vi "tt-钩外多胶检测-kA.vi"(9 "镜像产品角度":dbl=45.0, 11 "ImageSrc":T1(plugin-control)) -> (3 "ImgOut":T1(plugin-control))   [LabVIEW 2018]
uses:
  <vilib>/vision/Image Controls.llb/IMAQ Image.ctl
  <vilib>/vision/NI_Vision_Development_Module.lvlib
panel:
  out "error out":errorcluster
  out "Image Dst Out":T1
  in  "钩端向上部偏移量":dbl=100.0
  in  "Annulus":T2={"Center X"=0, "Center Y"=0, "Inner Radius"=27, "Outer Radius"=107, "Start Angle"=0.0, "End Angle"=0.0} {"End Angle" min=-90.0 max=90.0 step=1.0 format="%.2f"; "Start Angle" min=-90.0 max=90.0 step=1.0 format="%.2f"; "Center X" scale=0.0..1024.0}
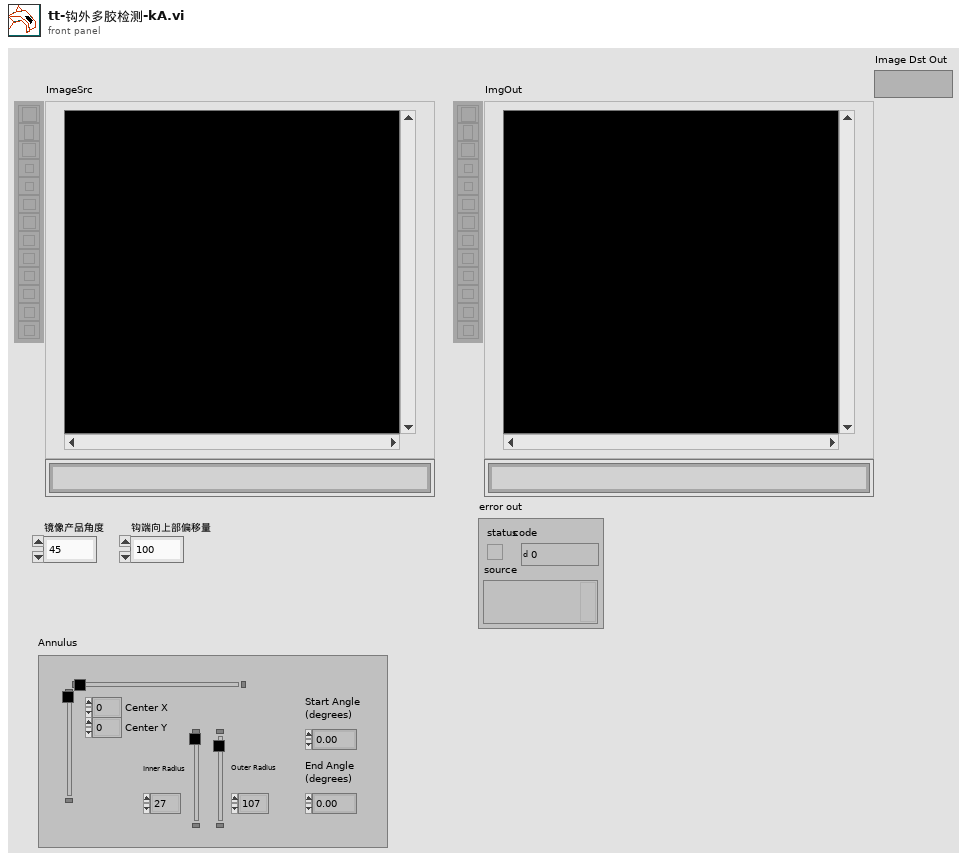
[diagram p1: front panel]
types:
  T1 = typedef "IMAQ Image.ctl" = refnum<image>
  T2 = typedef "IMAQ Circle" = cluster{"Center X":i32, "Center Y":i32, "Inner Radius":i32, "Outer Radius":i32, "Start Angle":dbl, "End Angle":dbl}
  T3 = typedef "Image Type" = u32
  T4 = typedef "ROI Descriptor" = cluster{"Global Rectangle":i32[], "Contours":cluster{"ID":enum32{"External", "Internal"}, "Type":u32, "Coordinates":i32[]}[]}
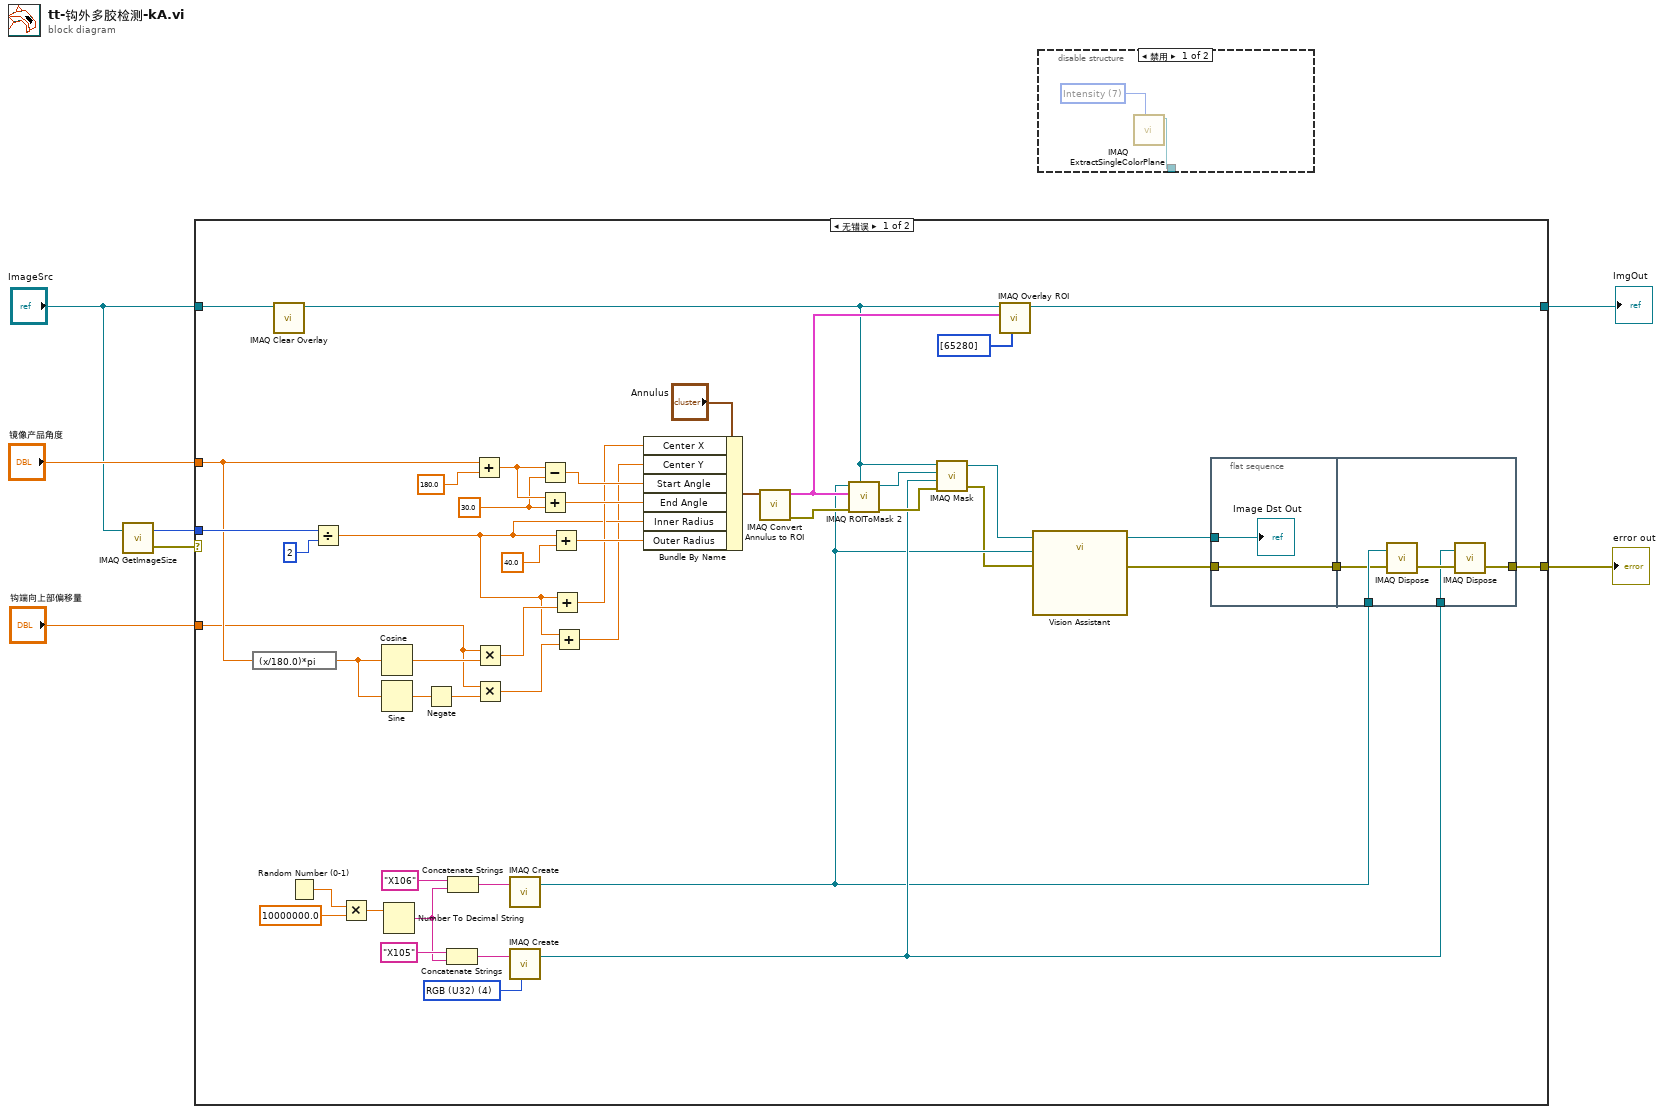
[diagram p0: block diagram]
diagram:
  n1 = call "IMAQ GetImageSize"("Image"="ImageSrc") -> ("Y Resolution"=w4:i32, "error out"=w5:errorcluster)  [unwired: 3 in, 1 out]
  n2 = case shown="无错误" w5 {
    selector: w5 -> [_ w62]
    tunnel: "镜像产品角度" -> [w43 _]
    tunnel: "ImageSrc" -> [w20 w63]
    tunnel: w4 -> [w47 _]
    tunnel: "钩端向上部偏移量" -> [w38 _]
    tunnel: [w29 w63] -> w2
    tunnel: [w15 w62] -> w1
    frame No Error {
      w16 = T3 4 items=["Grayscale (U8)", "Grayscale (I16)", "Grayscale (SGL)", "Complex (CSG)", "RGB (U32)", "HSL (U32)", "RGB (U64)", "Grayscale (U16)"] ("Image Type")
      w48 = 30.0 ("y")
      n3 = expression code="(x/180.0)*pi" ("角度转换至弧度")(w43) -> (w41:dbl)
      n4 = call "IMAQ Clear Overlay"("Image"=w20) -> ("Image Out"=w19:T1)  [unwired: 9 in, 1 out]
      n5 = Random Number (0-1)() -> (number: 0 to 1=w23:dbl)
      n6 = Divide(x=w47, y=2) -> (x/y=w34:dbl)
      n7 = Multiply(x=w23, y=10000000.0) -> (x*y=w25:dbl)
      n8 = Cosine(x=w41) -> (cos(x)=w40:dbl)
      n9 = Sine(x=w41) -> (sin(x)=w42:dbl)
      n10 = Number To Decimal String(number=w25) -> (decimal integer string=w22:string)  [unwired: 1 in]
      n11 = Negate(x=w42) -> (-x=w39:dbl)
      n12 = Concatenate Strings("X105" ("字符串"), w22) -> (w27:string)
      n13 = Concatenate Strings("X106" ("字符串"), w22) -> (w30:string)
      n14 = Add(x=w43, y=180.0) -> (x+y=w51:dbl)
      n15 = Multiply(x=w38, y=w40) -> (x*y=w37:dbl)
      n16 = Multiply(x=w38, y=w39) -> (x*y=w35:dbl)
      n17 = call "IMAQ Create"("Image Name"=w30) -> ("New Image"=w12:T1)  [unwired: 4 in, 1 out]
      n18 = call "IMAQ Create"("Image Name"=w27, "Image Type"=w16) -> ("New Image"=w14:T1)  [unwired: 3 in, 1 out]
      n19 = Subtract(x=w51, y=w48) -> (x-y=w50:dbl)
      n20 = Add(x=w51, y=w48) -> (x+y=w49:dbl)
      n21 = Add(x=w34, y=40.0) -> (x+y=w44:dbl)
      n22 = Add(x=w34, y=w37) -> (x+y=w36:dbl)
      n23 = Add(x=w34, y=w35) -> (x+y=w33:dbl)
      n24 = Bundle By Name(cluster="Annulus", "Center X"=w36, "Center Y"=w33, "Start Angle"=w50, "End Angle"=w49, "Inner Radius"=w34, "Outer Radius"=w44) -> (w53:T2)
      n25 = call "IMAQ Convert Annulus to ROI"("Annulus"=w53) -> ("error out"=w21:errorcluster, "ROI Descriptor"=w28:T4)  [unwired: 8 in]
      n26 = call "IMAQ ROIToMask 2"("Image Model"=w19, "error in (no error)"=w21, "ROI Descriptor"=w28, "Image"=w12) -> ("error out"=w17:errorcluster, "Image Out"=w18:T1)  [unwired: 5 in, 1 out]
      n27 = call "IMAQ Mask"("error in (no error)"=w17, "Image Dst"=w14, "Image Mask"=w18, "Image Src"=w19) -> ("error out"=w11:errorcluster, "Image Dst Out"=w13:T1)  [unwired: 1 in]
      n28 = call "IMAQ Overlay ROI"("Colors (Green)"=u32[] [65280], "ROI Descriptor"=w28, "Image"=w19) -> ("Image Out"=w29:T1)  [unwired: 7 in, 1 out]
      n29 = call "Vision Assistant"("Image In"=w13, "Image Dst"=w12, "error in"=w11) -> ("Image Out"=w8:T1, "error out"=w10:errorcluster)  [unwired: 23 in]
      n30 = flat-sequence {
        tunnel: w10 -> [w56]
        tunnel: [w56] -> w9
        tunnel: w8 -> [w55]
        tunnel: [w60] -> w15
        tunnel: w14 -> [w59]
        tunnel: w12 -> [w58]
        tunnel: w9 -> [w57]
        frame #0 {
          "Image Dst Out" <- w55
        }
        frame #1 {
          n31 = call "IMAQ Dispose"("Image"=w58, "error in (no error)"=w57) -> ("error out"=w61:errorcluster)  [unwired: 4 in]
          n32 = call "IMAQ Dispose"("Image"=w59, "error in (no error)"=w61) -> ("error out"=w60:errorcluster)  [unwired: 4 in]
        }
      }
    }
    frame Error {
    }
  }
  "ImgOut" <- w2
  "error out" <- w1
  n33 = disable-structure shown="禁用" {
    disable-tunnel: [w64 _] -> _
    frame Disabled {
      w65 = 7 items=["Red", "Green", "Blue", "Hue", "Saturation", "Luminance", "Value", "Intensity"] ("Color Plane")
      n34 = call "IMAQ ExtractSingleColorPlane"("Color Plane"=w65) -> ("Image Dst Out"=w64:T1)  [unwired: 9 in, 1 out]
    }
    frame Enabled {
    }
  }
